vi "Enqueue Message (Array).vi"(6 "Tableau Message prioritaire ?":bool[](array[boolean]), 8 "error in (no error)":T1 caption="entrée d'erreur (pas d'erreur)", 9 "Tableau de données de messages":variant[](array[variant]), 10 "Tableau de messages":string[](array[string]), 11 "File d'attente de messages":refnum<queue>) -> (0 "error out":T1 caption="sortie d'erreur", 3 "File d'attente de message dup.":refnum<queue>)   [LabVIEW 2020, in "Message Queue.lvlib"]
doc: "Pour un message normal, placer le message à la fin de la file d'attente. Pour un message prioritaire, l'ajouter au début de la file."
uses:
  Message Queue.lvlib
  Message Cluster.ctl
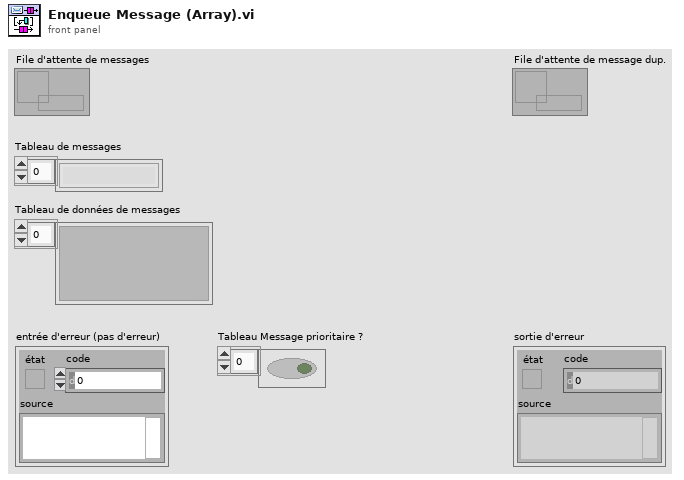
[diagram p1: front panel]
types:
  T1 = cluster{"état":bool, "code":i32, "source":string}
  T2 = typedef "Message Queue.lvlib/Message Cluster.ctl" = cluster{"Message":string, "Données de message":variant}
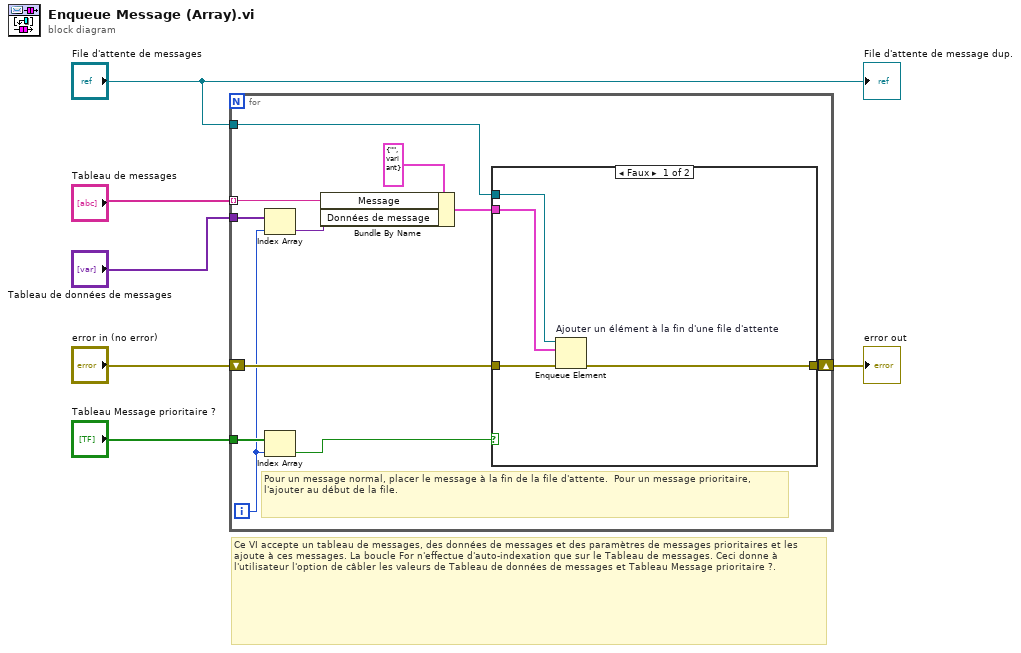
[diagram p0: block diagram]
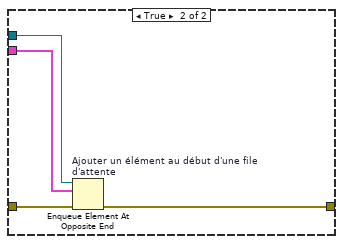
[diagram p2: hidden frame]
diagram:
  # "Ce VI accepte un tableau de messages, des données de messages et des paramètres de messages prioritaires et les ajoute à ces messages. La boucle For n'effectue d'auto-indexation que sur le Tableau de messages. Ceci donne à l'utilisateur l'option de câbler les valeurs de Tableau de données de messages et Tableau Message prioritaire ?."
  n1 = for {
    tunnel: "Tableau de messages" -> [w16] mode=indexing
    tunnel: "Tableau de données de messages" -> [w11]
    tunnel: "Tableau Message prioritaire ?" -> [w9]
    tunnel: "File d'attente de messages" -> [w13]
    shift-right: [w14] -> w2
    shift-left: "error in (no error)" -> [w15]
    i -> [w7]
    # "Pour un message normal, placer le message à la fin de la file d'attente.  Pour un message prioritaire, l'ajouter au début de la file."
    n2 = Index Array(array=w11, index=w7) -> (element=w10:variant)
    n3 = Index Array(array=w9, index=w7) -> (element=w8:bool)
    n4 = Bundle By Name(cluster=T2 {"Message"="", "Données de message"=variant} ("Message Cluster"), "Message"=w16, "Données de message"=w10) -> (w12:T2)
    n5 = case shown="Faux" w8 {
      tunnel: w15 -> [w21 w25]
      tunnel: [w20 w24] -> w14
      tunnel: w13 -> [w19 w23]
      tunnel: w12 -> [w18 w22]
      frame False {
        n6 = Enqueue Element "Ajouter un élément à la fin d'une file d'attente"(queue=w19, element=w18, error in (no error)=w21) -> (error out=w20:errorcluster)  [unwired: 1 in, 2 out]
      }
      frame True {
        n7 = Enqueue Element At Opposite End "Ajouter un élément au début d'une file d'attente"(queue=w23, element=w22, error in (no error)=w25) -> (error out=w24:errorcluster)  [unwired: 1 in, 2 out]
      }
    }
  }
  "error out" <- w2
  "File d'attente de message dup." <- "File d'attente de messages"
